vi "Error Query.vi"(8 "error in (no error)":errorcluster, 10 "Check cycles (11)":i32=11, 11 "VISA resource name":refnum<visa-resource-name>) -> (0 "error out":errorcluster, 1 "Error":bool, 2 "Error Message":string, 3 "VISA resource name out":refnum<visa-resource-name>)   [LabVIEW 2020, in "Datron D4xxx.lvlib"]
doc: "This VI checks for instrument RQS. It tries to check it every 100ms for at least \"Check cycles\" cycles. Defaultly it's set to 11 cycles (1.2 sec) because theese instruments are a bit lazy."
uses:
  Datron D4xxx.lvlib
panel:
  out "Last SRQ cycle":i32
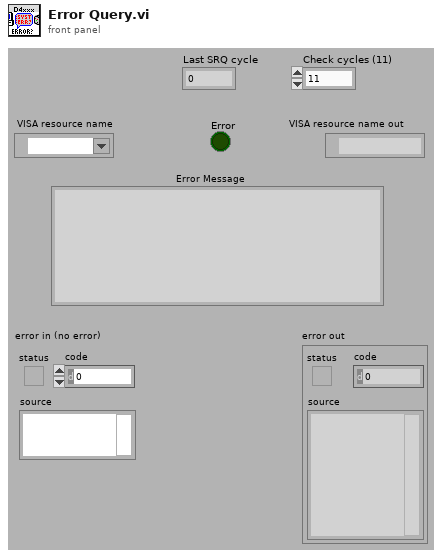
[diagram p1: front panel]
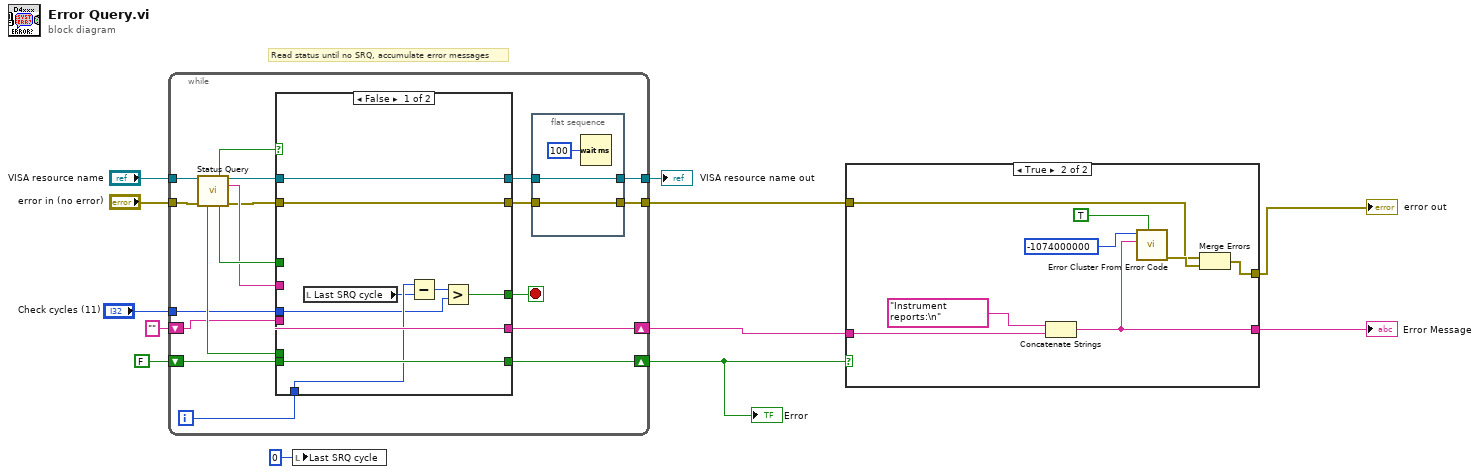
[diagram p0: block diagram]
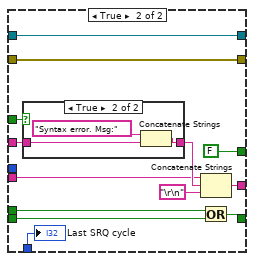
[diagram p2: hidden frame]
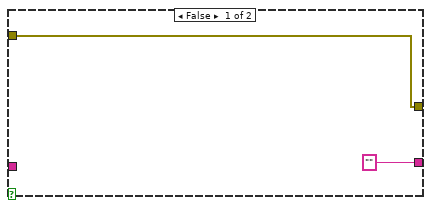
[diagram p4: hidden frame]
diagram:
  # "Read status until no SRQ, accumulate error messages"
  n1 = while {
    tunnel: "error in (no error)" -> [w31]
    tunnel: "VISA resource name" -> [w30]
    tunnel: [w17] -> w8
    tunnel: [w16] -> w7
    shift-right: [w26] -> w5
    shift-left: "" -> [w25]
    shift-right: [w24] -> w6
    shift-left: FALSE -> [w23]
    tunnel: "Check cycles (11)" -> [w13]
    i -> [w15]
    stop <- w14 stop-if-true
    n2 = call "Status Query.vi"("VISA resource name"=w30, "error in (no error)"=w31) -> ("SRQ"=w20:bool, "VISA resource name out"=w21:refnum<visa-resource-name>, "Measurement message"=w27:string, "Error"=w29:bool, "Syntax error"=w28:bool, "error out"=w22:errorcluster)  [unwired: 5 in, 3 out]
    n3 = case shown="False" w20 {
      tunnel: w29 -> [_ w56]
      tunnel: w28 -> [_ w55]
      tunnel: w27 -> [_ w54]
      tunnel: [w41 w52] -> w26
      tunnel: w25 -> [w41 w50]
      tunnel: [w40 w49] -> w24
      tunnel: w23 -> [w40 w48]
      tunnel: w22 -> [w43 w46]
      tunnel: [w43 w46] -> w19
      tunnel: w21 -> [w42 w47]
      tunnel: [w42 w47] -> w18
      tunnel: w15 -> [w39 w45]
      tunnel: [w36 FALSE] -> w14
      tunnel: w13 -> [w35 _]
      frame False {
        n4 = local read "Last SRQ cycle"() -> (w38:i32)
        n5 = Subtract(x=w39, y=w38) -> (x-y=w37:i32)
        n6 = Greater?(x=w37, y=w35) -> (0:w36:bool)
      }
      frame True {
        n7 = case shown="True" w55 {
          tunnel: w54 -> [w57 w59]
          tunnel: [w57 w58] -> w53
          frame False {
          }
          frame True {
            n8 = Concatenate Strings("Syntax error. Msg:" ("string"), w59) -> (w58:string)
          }
        }
        n9 = Concatenate Strings(w50, w53, "\r\n") -> (w52:string)
        n10 = Or(x=w56, y=w48) -> (x .or. y?=w49:bool)
        "Last SRQ cycle" <- w45
      }
    }
    n11 = flat-sequence {
      tunnel: [w34] -> w16
      tunnel: w19 -> [w34]
      tunnel: [w33] -> w17
      tunnel: w18 -> [w33]
      frame #0 {
        n12 = Wait (ms)(milliseconds to wait=u32 100) -> ()  [unwired: 1 out]
      }
    }
  }
  "VISA resource name out" <- w8
  "Error" <- w6
  n13 = local write "Last SRQ cycle"(0 ("Last no SRQ cycle")) -> ()
  n14 = case shown="True" w6 {
    tunnel: [w61 w65] -> w12
    tunnel: w5 -> [_ w67]
    tunnel: ["" w64] -> w11
    tunnel: w7 -> [w61 w63]
    frame False {
    }
    frame True {
      n15 = Concatenate Strings("Instrument reports:\n" ("Source"), w67) -> (w64:string)
      n16 = call <vilib>:"Error Cluster From Error Code.vi"("show call chain? (False)"=TRUE, "error message (\"\")"=w64, "error code (0)"=-1074000000 ("Code")) -> ("error out"=w66:errorcluster)  [unwired: 6 in]
      n17 = Merge Errors(w63, w66) -> (w65:errorcluster)
    }
  }
  "error out" <- w12
  "Error Message" <- w11
